vi "find running app.vi"() -> ()   [LabVIEW 2010]
uses:
  file/file action.ctl
panel:
  out "Launching an application":bool
  out "found app":path
  out "app names":string[](array[string])
  out "file names":string[](array[string])
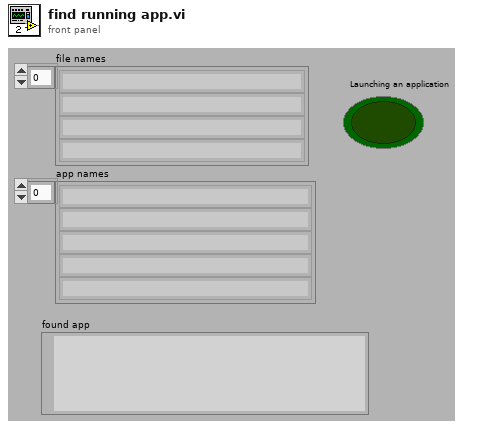
[diagram p1: front panel]
types:
  T1 = typedef "file action.ctl" = enum16{"Save", "Open"}
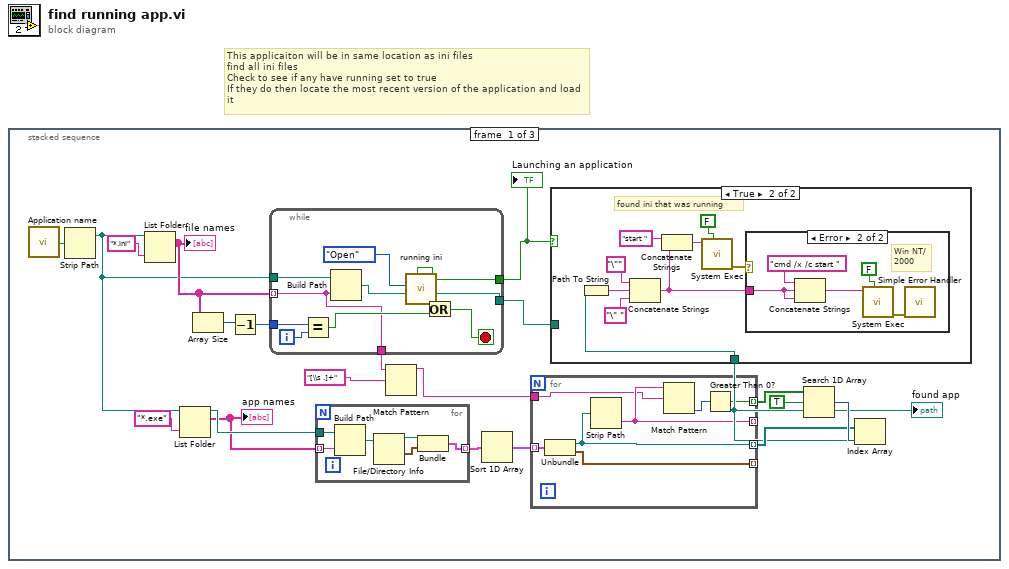
[diagram p0: block diagram]
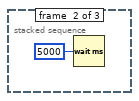
[diagram p4: hidden frame]
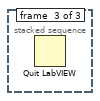
[diagram p5: hidden frame]
diagram:
  # "This applicaiton will be in same location as ini files\nfind all ini files\nCheck to see if any have running set to true\nIf they do then locate the most recent version of the application and load it"
  n1 = stacked-sequence {
    frame #0 {
      n2 = call "Application name.vi"() -> ("Ini file path"=w21:path)  [unwired: 4 in, 3 out]
      n3 = Strip Path(path=w21) -> (stripped path=w13:path)  [unwired: 1 out]
      n4 = List Folder(path=w13, pattern="*.ini") -> (filenames=w19:string[])  [unwired: 2 in, 3 out]
      "file names" <- w19
      n5 = List Folder(path=w13, pattern="*.exe") -> (path out=w12:path, filenames=w11:string[])  [unwired: 2 in, 2 out]
      "app names" <- w11
      n6 = Array Size(array=w19) -> (size(s)=w18:i32)
      n7 = Decrement(x=w18) -> (x-1=w17:i32)
      n8 = while {
        tunnel: w13 -> [w57]
        tunnel: w19 -> [w49] mode=indexing
        tunnel: w17 -> [w54]
        tunnel: [w51] -> w16
        tunnel: [w50] -> w15
        tunnel: [w49] -> w8
        i -> [w55]
        stop <- w52 stop-if-true
        n9 = Equal?(x=w54, y=w55) -> (x = y?=w53:bool)
        n10 = Build Path(base path=w57, name or relative path=w49) -> (appended path=w50:path)
        n11 = call "running ini.vi"("Action"=file_action."Open", "Ini file path"=w50) -> ("running out"=w51:bool)  [unwired: 4 in]
        n12 = Or(x=w51, y=w53) -> (x .or. y?=w52:bool)
      }
      "Launching an application" <- w16
      n13 = for {
        tunnel: w12 -> [w34]
        tunnel: w11 -> [w33] mode=indexing
        tunnel: [w29] -> w10 mode=indexing
        n14 = Build Path(base path=w34, name or relative path=w33) -> (appended path=w32:path)
        n15 = File/Directory Info(path=w32) -> (path out=w31:path, last mod=w30:timestamp)  [unwired: 1 in, 5 out]
        n16 = Bundle("dup path"=w31, "last mod"=w30) -> (w29:cluster{"dup path":path, "last mod":timestamp})  [unwired: 1 in]
      }
      n17 = Match Pattern(string=w8, regular expression="[\\s .]+") -> (before substring=w6:string)  [unwired: 1 in, 3 out]
      n18 = Sort 1D Array(array=w10) -> (sorted array=w9:cluster{"dup path":path, "last mod":timestamp}[])
      n19 = for {
        tunnel: w9 -> [w28] mode=indexing
        tunnel: [w25] -> _ mode=indexing
        tunnel: [w27] -> w2 mode=indexing
        tunnel: [w26] -> _ mode=indexing
        tunnel: w6 -> [w24]
        tunnel: [w22] -> w5 mode=indexing
        n20 = Unbundle(w28) -> ("dup path"=w27:path, "last mod"=w26:timestamp)
        n21 = Strip Path(path=w27) -> (name=w25:string)  [unwired: 1 out]
        n22 = Match Pattern(string=w25, regular expression=w24) -> (offset past match=w23:i32)  [unwired: 1 in, 3 out]
        n23 = Greater Than 0?(x=w23) -> (x > 0?=w22:bool)
      }
      n24 = Search 1D Array(1D array=w5, element=TRUE) -> (index of element=w3:i32)  [unwired: 1 in]
      n25 = Index Array(array=w2, index=w3) -> (element=w1:path)
      "found app" <- w1
      n26 = case shown="True" w16 {
        tunnel: w15 -> [_ _]
        tunnel: w1 -> [_ w35]
        frame False {
          # "no ini. files had a running application"
        }
        frame True {
          # "found ini that was running"
          n27 = Path To String(path=w35) -> (string=w36:string)
          n28 = Concatenate Strings("\"" ("Substring"), w36, "\" " ("Substring")) -> (w38:string)
          n29 = Concatenate Strings("start " ("Substring"), w38) -> (w39:string)
          n30 = call <vilib>:"System Exec.vi"("wait until completion? (T)"=FALSE ("Wait until done"), "command line"=w39) -> ("error out"=w40:errorcluster)  [unwired: 6 in, 3 out]
          n31 = case shown="Error" w40 {
            tunnel: w38 -> [_ w44]
            frame No Error {
              # "Win 95/98/Me"
            }
            frame Error {
              # "Win NT/\n2000"
              n32 = Concatenate Strings("cmd /x /c start ", w44, w44) -> (w46:string)
              n33 = call <vilib>:"System Exec.vi"("wait until completion? (T)"=FALSE ("Wait until done"), "command line"=w46) -> ("error out"=w45:errorcluster)  [unwired: 6 in, 3 out]
              n34 = call <vilib>:"Simple Error Handler.vi"("error in (no error)"=w45) -> ()  [unwired: 4 in, 5 out]
            }
          }
        }
      }
    }
    frame #1 {
      n35 = Wait (ms)(milliseconds to wait=u32 5000) -> ()  [unwired: 1 out]
    }
    frame #2 {
      n36 = Quit LabVIEW() -> ()  [unwired: 1 in]
    }
  }
